vi "Test Mutex.vi"() -> ()   [LabVIEW 2013]
uses:
  <vilib>/LabVIEW Open Source Project/MQTT Control Packets/Control Packets/ControlPacket/Control Packet Type -- enum.ctl
  <vilib>/LabVIEW Open Source Project/MQTT Control Packets/Control Packets/ControlPacket/ControlPacket.lvclass
  <vilib>/LabVIEW Open Source Project/MQTT Control Packets/Control Packets/PUBLISH/PUBLISH.lvclass
  source/Client class/Client.lvclass
  <vilib>/LabVIEW Open Source Project/MQTT Connection/MQTT_Base/Base Class/MQTT_Base.lvclass
  <vilib>/LabVIEW Open Source Project/MQTT Connection/MQTT_Connection/Connection/Connection.lvclass
  <vilib>/LabVIEW Open Source Project/MQTT TCP Connection/MQTT_TCP/Connection/TCPConnection.lvclass
  <vilib>/LabVIEW Open Source Project/MQTT Control Packets/Control Packets/CONNACK/CONNACK.lvclass
panel:
  out "Array 2":string[](array[string])
  out "Array":T1[](array[typedef])
  out "server connected":bool
  out "listener error":errorcluster
  out "server session error":errorcluster
  out "error out":errorcluster
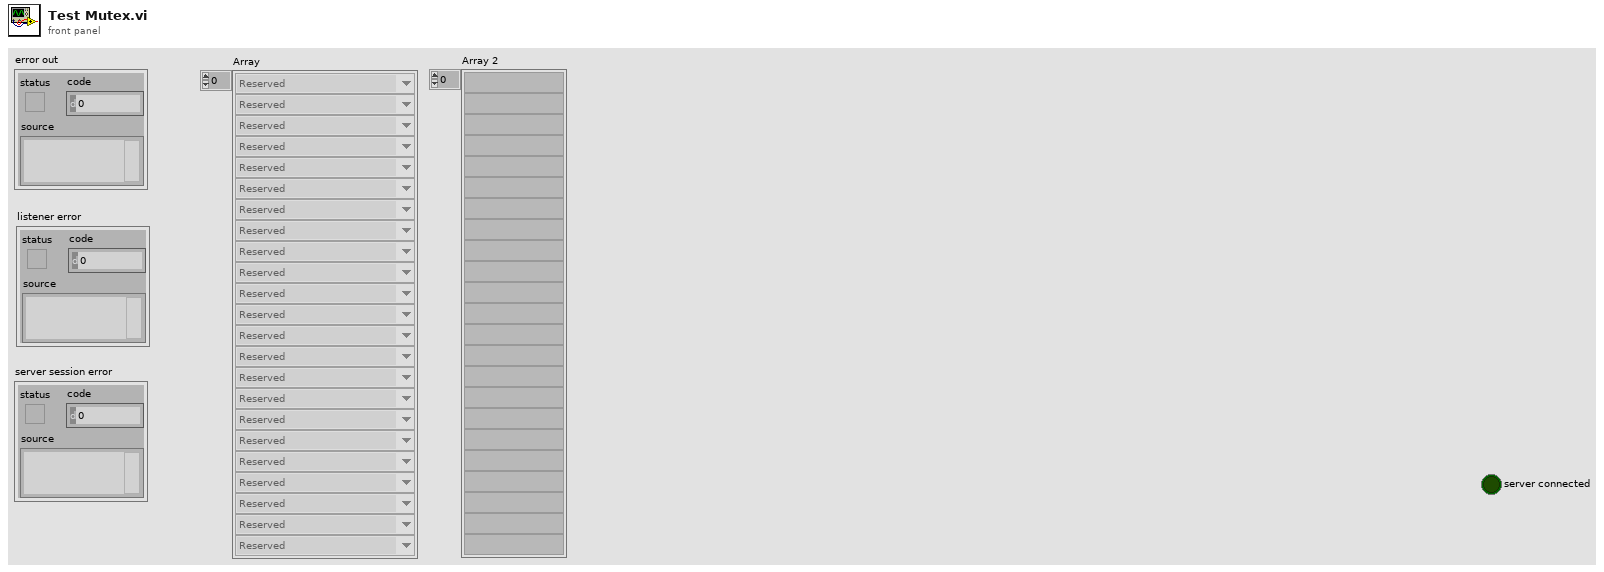
[diagram p1: front panel]
types:
  T1 = typedef "MQTT_Control_Packets.lvlib/ControlPacket.lvclass/Control Packet Type -- enum.ctl" = enum16{"Reserved", "CONNECT", "CONNACK", "PUBLISH", "PUBACK", "PUBREC", "PUBREL", "PUBCOMP", "SUBSCRIBE", "SUBACK", "UNSUBSCRIBE", "UNSUBACK", "PINGREQ", "PINGRESP", "DISCONNECT", "AUTH"}
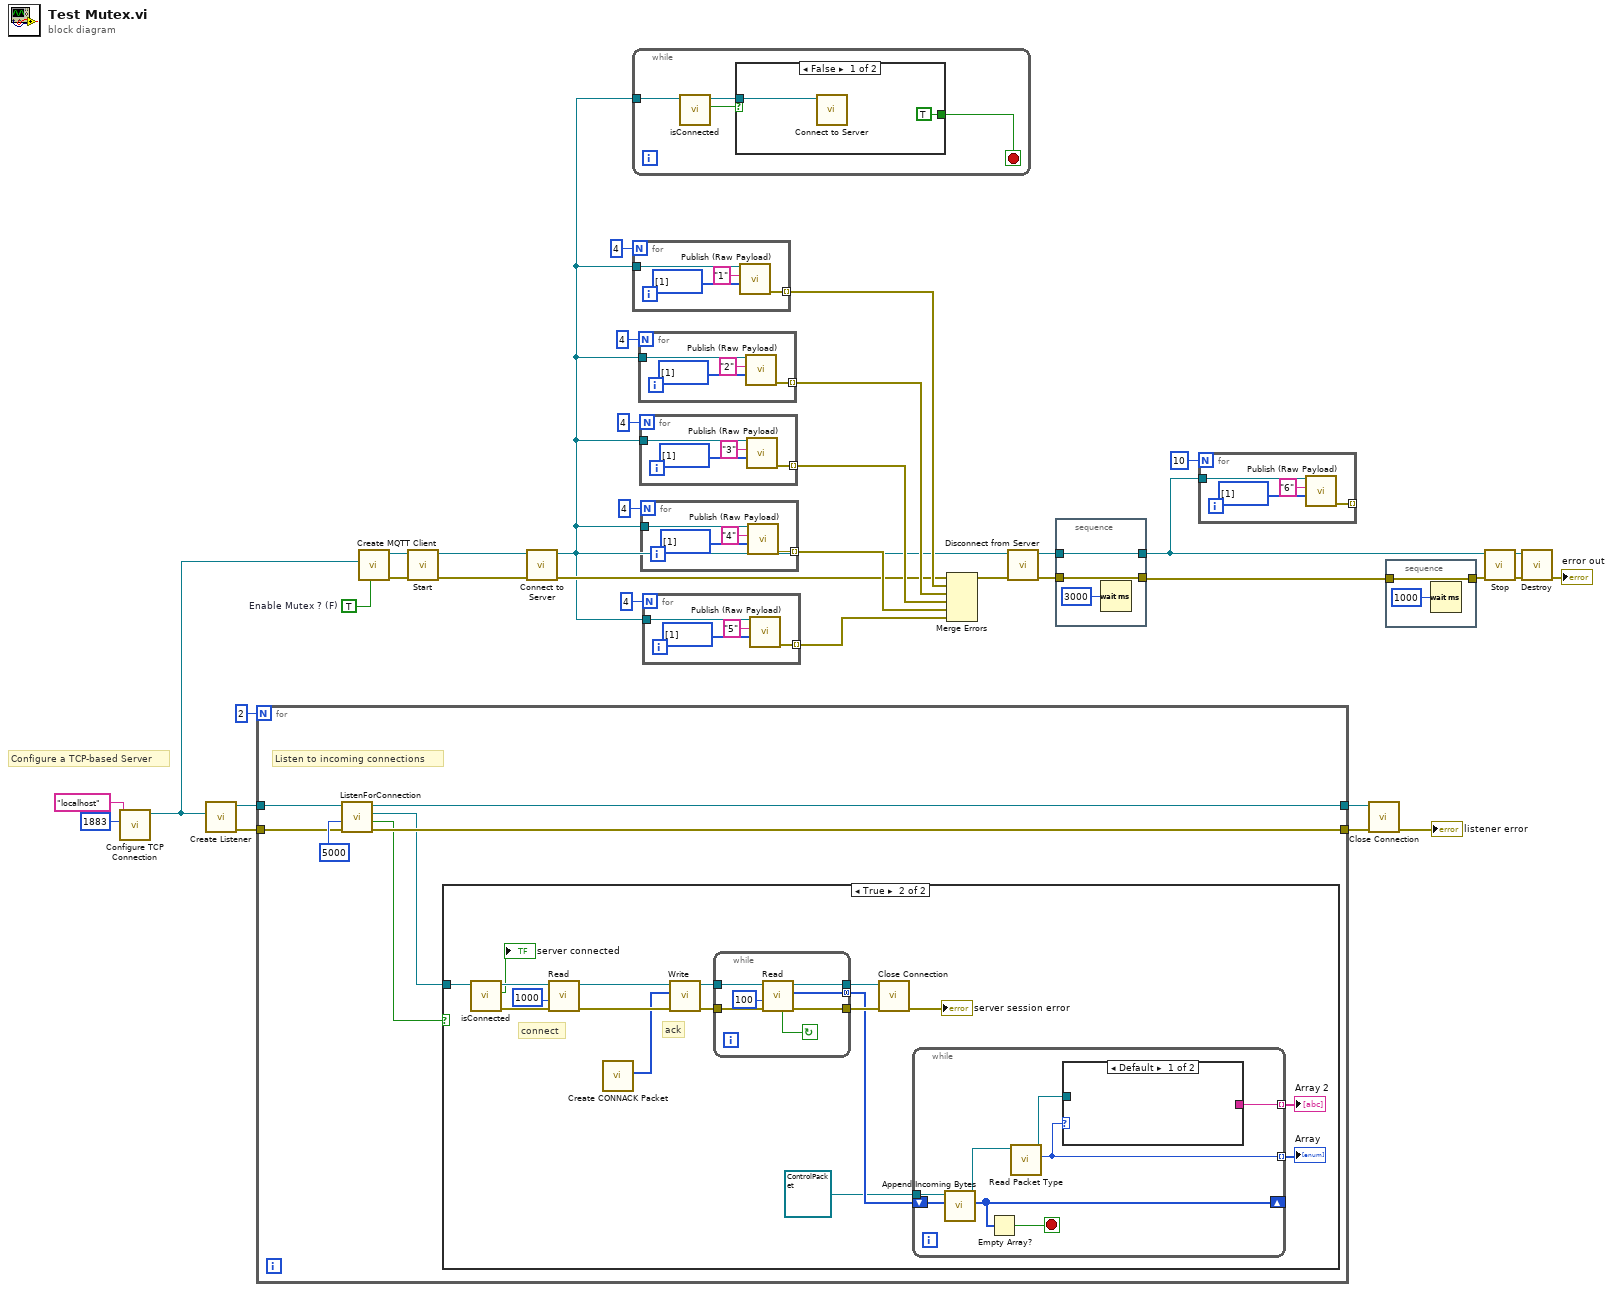
[diagram p0: block diagram]
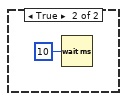
[diagram p2: hidden frame]
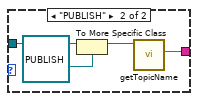
[diagram p4: hidden frame]
diagram:
  w20 = TRUE  # Enable Mutex ? (F)
  # "Configure a TCP-based Server"
  n1 = call <vilib>:"Configure TCP Connection.vi"("remote port (80)"=u16 1883, "address (localhost)"="localhost") -> ("TCPConnection"=w22:refnum<class "TCPConnection.lvclass">)  [unwired: 8 in, 1 out]
  n2 = call <vilib>:"Create Listener.vi"("Connection Configuration"=w22) -> ("error out"=w27:errorcluster, "Listener"=w29:refnum<class "Connection.lvclass">)  [unwired: 9 in]
  n3 = for {
    N: 2 -> [_]
    tunnel: w29 -> [w43]
    tunnel: [w41] -> w28
    tunnel: w27 -> [w40]
    tunnel: [w39] -> w26
    # "Listen to incoming connections"
    n4 = call <vilib>:"ListenForConnection.vi"("error in (no error)"=w40, "timeout (2000 ms)"=5000 ("bytes to read (100)"), "Listener"=w43) -> ("error out"=w39:errorcluster, "New connection"=w37:bool, "Connection"=w38:refnum<class "Connection.lvclass">, "Listener out"=w41:refnum<class "Connection.lvclass">)  [unwired: 5 in]
    n5 = case shown="True" w37 {
      tunnel: w38 -> [_ w56]
      frame False {
      }
      frame True {
        # "ack"
        # "connect"
        n6 = call <vilib>:"isConnected.vi"("Connection in"=w56) -> ("error out"=w54:errorcluster, "connected"=→"server connected":bool, "Connection out"=w55:refnum<class "Connection.lvclass">)  [unwired: 8 in]
        n7 = call <vilib>:"Read.vi"("error in (no error)"=w54, "timeout (2000 ms)"=1000 ("bytes to read (100)"), "TCPConnection in"=w55) -> ("error out"=w58:errorcluster, "TCPConnection out"=w59:refnum<class "Connection.lvclass">)  [unwired: 4 in, 3 out]
        n8 = call <vilib>:"Create CONNACK Packet.vi"() -> ("Bytes Stream"=w52:u8[])  [unwired: 9 in, 2 out]
        n9 = call <vilib>:"Write.vi"("error in (no error)"=w58, "Bytes"=w52, "Connection in"=w59) -> ("error out"=w50:errorcluster, "Connection"=w51:refnum<class "Connection.lvclass">)  [unwired: 7 in]
        n10 = while {
          tunnel: w51 -> [w78]
          tunnel: w50 -> [w77]
          tunnel: [w76] -> w49
          tunnel: [w75] -> w48
          tunnel: [w74] -> w47 mode=concatenating
          stop <- w73 continue-if-true
          n11 = call <vilib>:"Read.vi"("error in (no error)"=w77, "timeout (2000 ms)"=100 ("bytes to read (100)"), "TCPConnection in"=w78) -> ("error out"=w75:errorcluster, "Bytes"=w74:u8[], "TCPConnection out"=w76:refnum<class "Connection.lvclass">, "connected"=w73:bool)  [unwired: 4 in, 1 out]
        }
        n12 = call <vilib>:"Close Connection.vi"("error in (no error)"=w48, "Connection in"=w49) -> ("error out"=→"server session error":errorcluster)  [unwired: 8 in, 1 out]
        n13 = while {
          tunnel: refnum<class "ControlPacket.lvclass"> refnum ("Incomplete ControlPacket") -> [w67]
          shift-right: [w66] -> _
          shift-left: w47 -> [w68]
          tunnel: [w63] -> w45 mode=indexing
          tunnel: [w61] -> w44 mode=indexing
          stop <- w65 stop-if-true
          n14 = call <vilib>:"Append Incoming Bytes.vi"("Incoming Packets"=w68, "Incomplete ControlPacket"=w67) -> ("Remaining Packets"=w66:u8[], "ControlPacket"=w64:refnum<class "ControlPacket.lvclass">)  [unwired: 6 in, 2 out]
          n15 = Empty Array?(array=w66) -> (empty?=w65:bool)
          n16 = call <vilib>:"Read Packet Type.vi"("ControlPacket in"=w64) -> ("Control Packet Type"=w63:T1, "ControlPacket out"=w62:refnum<class "ControlPacket.lvclass">)  [unwired: 9 in]
          n17 = case shown="Default" w63 {
            tunnel: w62 -> [_ w72]
            tunnel: [_ w69] -> w61
            frame Default {
            }
            frame "PUBLISH" {
              n18 = To More Specific Class(target class=refnum<class "PUBLISH.lvclass"> refnum ("PUBLISH in"), reference=w72) -> (specific class reference=w71:refnum<class "PUBLISH.lvclass">)  [unwired: 1 in, 1 out]
              n19 = call <vilib>:"getTopicName.vi"("PUBLISH in"=w71) -> ("Topic"=w69:string)  [unwired: 8 in, 2 out]
            }
          }
        }
        "Array" <- w45
        "Array 2" <- w44
      }
    }
  }
  n20 = call "Create MQTT Client.vi"("Enable Mutex ? (F)"=w20, "Connection Configuration"=w22) -> ("error out"=w35:errorcluster, "Client out"=w33:refnum<class "Client.lvclass">)  [unwired: 8 in]
  n21 = call <vilib>:"Start.vi"("error in (no error)"=w35, "MQTT_Base in"=w33) -> ("error out"=w34:errorcluster, "MQTT_Base out"=w32:refnum<class "Client.lvclass">)  [unwired: 7 in, 1 out]
  n22 = call "Connect to Server.vi"("error in (no error)"=w34, "Client in"=w32) -> ("error out"=w8:errorcluster, "Client out"=w7:refnum<class "Client.lvclass">)  [unwired: 6 in, 2 out]
  n23 = while {
    tunnel: w7 -> [w83]
    stop <- w80 stop-if-true
    n24 = call <vilib>:"isConnected.vi"("Client in"=w83) -> ("connected"=w82:bool, "Client out"=w81:refnum<class "Client.lvclass">)  [unwired: 8 in, 1 out]
    n25 = case shown="False" w82 {
      tunnel: w81 -> [w85 _]
      tunnel: [TRUE _] -> w80
      frame False {
        n26 = call "Connect to Server.vi"("Client in"=w85) -> ()  [unwired: 7 in, 4 out]
      }
      frame True {
        n27 = Wait (ms)(milliseconds to wait=u32 10) -> ()  [unwired: 1 out]
      }
    }
  }
  n28 = for {
    N: 4 -> [_]
    tunnel: w7 -> [w88]
    tunnel: [w87] -> w9 mode=indexing
    n29 = call "Publish (Raw Payload).vi"("Binary Payload"=u8[] [1], "Topic Name"="1", "Client in"=w88) -> ("error out"=w87:errorcluster)  [unwired: 6 in, 2 out]
  }
  n30 = for {
    N: 4 -> [_]
    tunnel: w7 -> [w92]
    tunnel: [w91] -> w10 mode=indexing
    n31 = call "Publish (Raw Payload).vi"("Binary Payload"=u8[] [1], "Topic Name"="2", "Client in"=w92) -> ("error out"=w91:errorcluster)  [unwired: 6 in, 2 out]
  }
  n32 = for {
    N: 4 -> [_]
    tunnel: w7 -> [w96]
    tunnel: [w95] -> w11 mode=indexing
    n33 = call "Publish (Raw Payload).vi"("Binary Payload"=u8[] [1], "Topic Name"="3", "Client in"=w96) -> ("error out"=w95:errorcluster)  [unwired: 6 in, 2 out]
  }
  n34 = for {
    N: 4 -> [_]
    tunnel: w7 -> [w100]
    tunnel: [w99] -> w13 mode=indexing
    n35 = call "Publish (Raw Payload).vi"("Binary Payload"=u8[] [1], "Topic Name"="4", "Client in"=w100) -> ("error out"=w99:errorcluster)  [unwired: 6 in, 2 out]
  }
  n36 = for {
    N: 4 -> [_]
    tunnel: w7 -> [w104]
    tunnel: [w103] -> w12 mode=indexing
    n37 = call "Publish (Raw Payload).vi"("Binary Payload"=u8[] [1], "Topic Name"="5", "Client in"=w104) -> ("error out"=w103:errorcluster)  [unwired: 6 in, 2 out]
  }
  n38 = Merge Errors(w8, w9, w10, w11, w13, w12) -> (w19:errorcluster)
  n39 = call "Disconnect from Server.vi"("error in (no error)"=w19, "Client in"=w7) -> ("error out"=w21:errorcluster, "Client out"=w1:refnum<class "Client.lvclass">)  [unwired: 7 in, 1 out]
  n40 = stacked-sequence {
    tunnel: w21 -> [w108]
    tunnel: [w108] -> w3
    tunnel: [w107] -> w2
    tunnel: w1 -> [w107]
    frame #0 {
      n41 = Wait (ms)(milliseconds to wait=u32 3000) -> ()  [unwired: 1 out]
    }
  }
  n42 = for {
    N: 10 -> [_]
    tunnel: w2 -> [w111]
    tunnel: [w110] -> _ mode=indexing
    n43 = call "Publish (Raw Payload).vi"("Binary Payload"=u8[] [1], "Topic Name"="6", "Client in"=w111) -> ("error out"=w110:errorcluster)  [unwired: 6 in, 2 out]
  }
  n44 = call <vilib>:"Close Connection.vi"("error in (no error)"=w26, "Connection in"=w28) -> ("error out"=→"listener error":errorcluster)  [unwired: 8 in, 1 out]
  n45 = stacked-sequence {
    tunnel: w3 -> [w114]
    tunnel: [w114] -> w4
    frame #0 {
      n46 = Wait (ms)(milliseconds to wait=u32 1000) -> ()  [unwired: 1 out]
    }
  }
  n47 = call <vilib>:"Stop.vi"("error in (no error)"=w4, "MQTT_Base in"=w2) -> ("error out"=w30:errorcluster, "MQTT_Base out"=w31:refnum<class "Client.lvclass">)  [unwired: 7 in, 1 out]
  n48 = call <vilib>:"Destroy.vi"("error in (no error)"=w30, "MQTT_Base in"=w31) -> ("error out"=→"error out":errorcluster)  [unwired: 8 in, 1 out]
